vi "Read Write LS DAS App Config.vi"(7 "Write (F)":bool, 8 "Error IN":errorcluster, 10 "LS DAS Config":T1={"Location"="", "Profiles Path"=path "", "Current Profile"="", "CA Number"="", "Cycles Completed"=0, "Stagger Time (ms)"=0, "Pumps Present"={"Pump 1"=FALSE, "Pump 2"=FALSE, "Pump 3"=FALSE, "Pump 4"=FALSE, "Pump 5"=FALSE, "Pump 6"=FALSE}, "Data Log Init"={"Data Path"=path "", "Data Log Rate (S/s)"=0, "AKLH Rate (Hours/S)"=0.0, "Sync Time Offset (min)"=0, "IP Last 3"=0, "WebDAV IP"=""}, "Email Handler IP"="", "Cycle Threshold:"=3.0, "Cycle Pts to Avg:"=3, "Anomaly Threshold:"=3.0, "Normal Steps:"=3, "Step Threshold:"=3.0, "Bank 1 Offset"=0.0, "Bank 2 Offset"=0.0, "LS Power (Freq):"=0.0, "LS Power (Duty):"=0.0, "Bank 1 Present"={"1"=FALSE, "2"=FALSE, "3"=FALSE, "4"=FALSE, "5"=FALSE}, "Bank 2 Present"={"6"=FALSE, "7"=FALSE, "8"=FALSE, "9"=FALSE, "10"=FALSE}, "Data File Name"="", "Detection Mode"=0, "Serial Numbers"=[], "Profile Record"=FALSE, "Bank2 Record Rate"=0} {"Bank2 Record Rate" step=1; "Detection Mode" min=0 max=999999 step=1; "LS Power (Duty):" min=0.0 max=999999.0 step=1.0; "LS Power (Freq):" min=0.0 max=999999.0 step=1.0; "Bank 2 Offset" min=0.0 max=999999.0 step=1.0; "Bank 1 Offset" min=0.0 max=999999.0 step=1.0; "Step Threshold:" max=999999.0 step=1.0; "Normal Steps:" max=999999 step=1; "Anomaly Threshold:" max=999999.0 step=1.0; "Cycle Pts to Avg:" min=0 max=999999 step=1; "Cycle Threshold:" min=0.0 max=999999.0 step=1.0}, 11 "Refnum in":T3) -> (0 "Error OUT":errorcluster, 2 "LS DAS Config OUT":T1={"Location"="", "Profiles Path"=path "", "Current Profile"="", "CA Number"="", "Cycles Completed"=0, "Stagger Time (ms)"=0, "Pumps Present"={"Pump 1"=FALSE, "Pump 2"=FALSE, "Pump 3"=FALSE, "Pump 4"=FALSE, "Pump 5"=FALSE, "Pump 6"=FALSE}, "Data Log Init"={"Data Path"=path "", "Data Log Rate (S/s)"=0, "AKLH Rate (Hours/S)"=0.0, "Sync Time Offset (min)"=0, "IP Last 3"=0, "WebDAV IP"=""}, "Email Handler IP"="", "Cycle Threshold:"=3.0, "Cycle Pts to Avg:"=3, "Anomaly Threshold:"=3.0, "Normal Steps:"=3, "Step Threshold:"=3.0, "Bank 1 Offset"=0.0, "Bank 2 Offset"=0.0, "LS Power (Freq):"=0.0, "LS Power (Duty):"=0.0, "Bank 1 Present"={"1"=FALSE, "2"=FALSE, "3"=FALSE, "4"=FALSE, "5"=FALSE}, "Bank 2 Present"={"6"=FALSE, "7"=FALSE, "8"=FALSE, "9"=FALSE, "10"=FALSE}, "Data File Name"="", "Detection Mode"=0, "Serial Numbers"=[], "Profile Record"=FALSE, "Bank2 Record Rate"=0} {"Bank2 Record Rate" step=1; "Detection Mode" min=0 max=999999 step=1; "LS Power (Duty):" min=0.0 max=999999.0 step=1.0; "LS Power (Freq):" min=0.0 max=999999.0 step=1.0; "Bank 2 Offset" min=0.0 max=999999.0 step=1.0; "Bank 1 Offset" min=0.0 max=999999.0 step=1.0; "Step Threshold:" max=999999.0 step=1.0; "Normal Steps:" max=999999 step=1; "Anomaly Threshold:" max=999999.0 step=1.0; "Cycle Pts to Avg:" min=0 max=999999 step=1; "Cycle Threshold:" min=0.0 max=999999.0 step=1.0}, 3 "Refnum out":T3)   [LabVIEW 2018]
uses:
  <vilib>/Utility/config.llb/Config Data RefNum.ctl
  Type Defs/LS DAS App Config.ctl
  Data Logger/Data Log Init.ctl
  <vilib>/Utility/config.llb/NI_LVConfig.lvlib
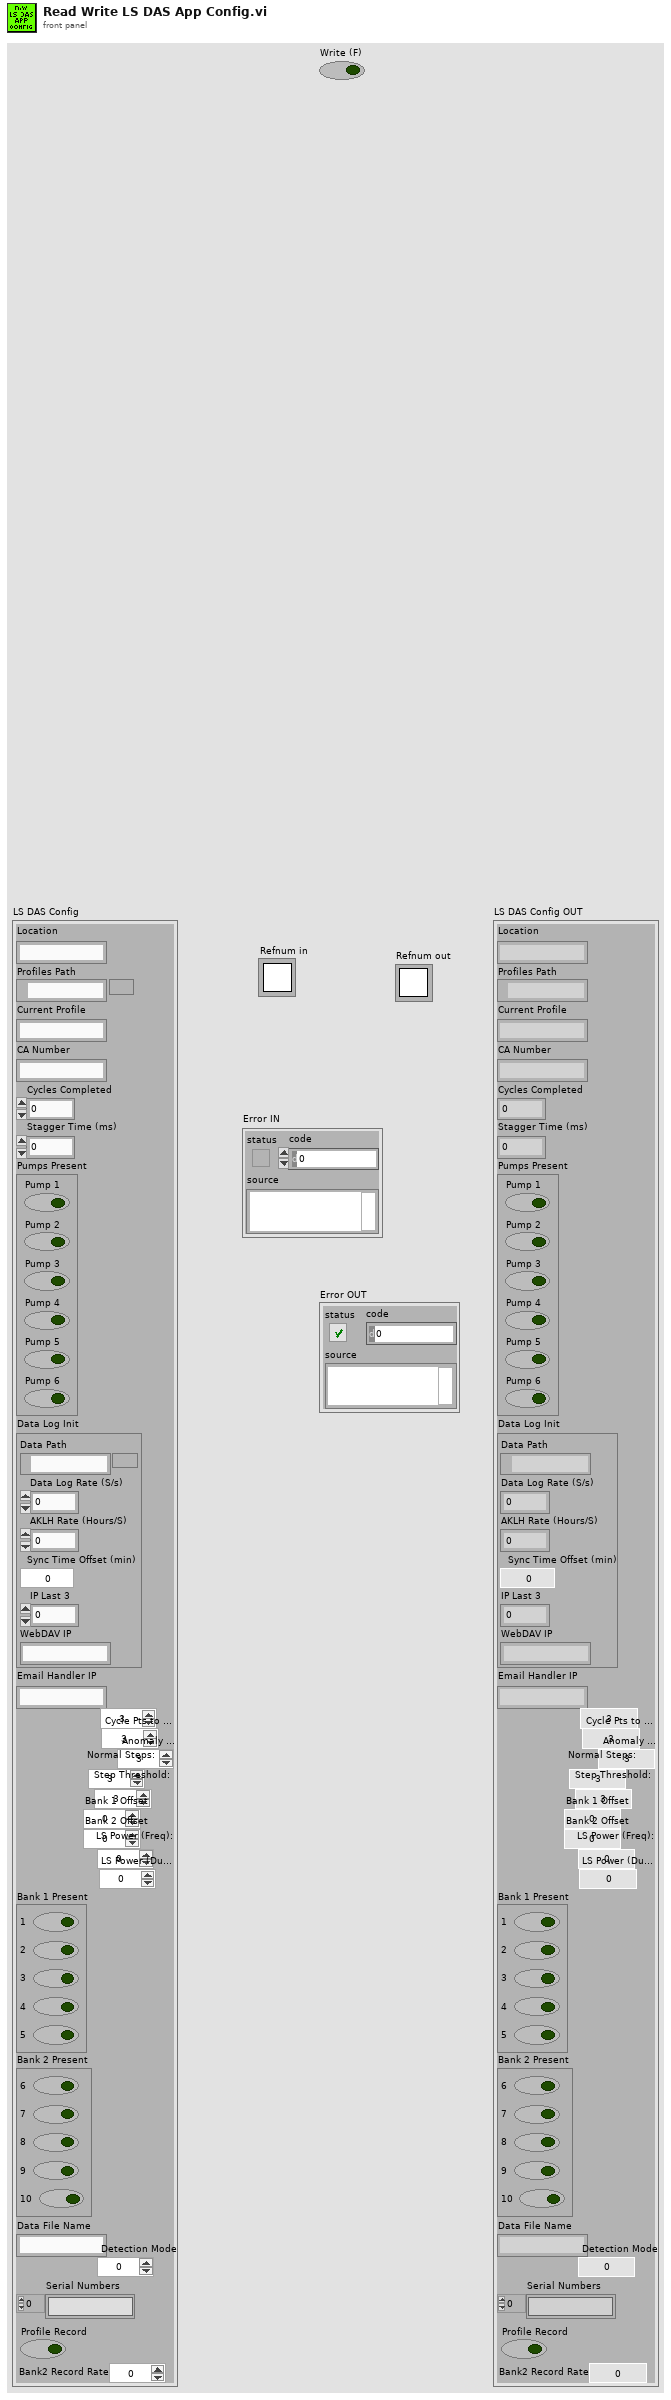
[diagram p1: front panel]
types:
  T1 = typedef "LS DAS App Config.ctl" = cluster{"Location":string, "Profiles Path":path, "Current Profile":string, "CA Number":string, "Cycles Completed":u32, "Stagger Time (ms)":i32, "Pumps Present":cluster{"Pump 1":bool, "Pump 2":bool, "Pump 3":bool, "Pump 4":bool, "Pump 5":bool, "Pump 6":bool}, "Data Log Init":T2, "Email Handler IP":string, "Cycle Threshold:":dbl, "Cycle Pts to Avg:":i32, "Anomaly Threshold:":dbl, "Normal Steps:":u32, "Step Threshold:":dbl, "Bank 1 Offset":dbl, "Bank 2 Offset":dbl, "LS Power (Freq):":dbl, "LS Power (Duty):":dbl, "Bank 1 Present":cluster{"1":bool, "2":bool, "3":bool, "4":bool, "5":bool}, "Bank 2 Present":cluster{"6":bool, "7":bool, "8":bool, "9":bool, "10":bool}, "Data File Name":string, "Detection Mode":i32, "Serial Numbers":string[], "Profile Record":bool, "Bank2 Record Rate":u16}
  T2 = typedef "Data Log Init.ctl" = cluster{"Data Path":path, "Data Log Rate (S/s)":u32, "AKLH Rate (Hours/S)":dbl, "Sync Time Offset (min)":i32, "IP Last 3":i32, "WebDAV IP":string}
  T3 = typedef "NI_LVConfig.lvlib/Config Data RefNum.ctl" = refnum<k1>
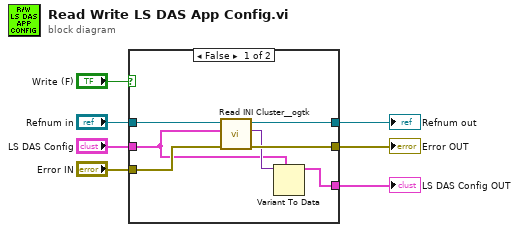
[diagram p0: block diagram]
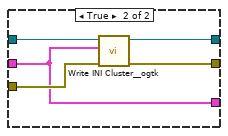
[diagram p2: hidden frame]
diagram:
  n1 = case shown="False" "Write (F)" {
    tunnel: "Refnum in" -> [w14 w19]
    tunnel: "LS DAS Config" -> [w10 w16]
    tunnel: "Error IN" -> [w13 w18]
    tunnel: [w8 w17] -> w4
    tunnel: [w9 w16] -> w1
    tunnel: [w12 w15] -> w5
    frame False {
      n2 = call <userlib>:"Read INI Cluster__ogtk.vi"("error in (no error)"=w13, "INI Fomatted Cluster Type"=w10, "refnum"=w14) -> ("error out"=w12:errorcluster, "INI Fomatted Cluster"=w11:variant, "dup refnum"=w8:T3)  [unwired: 4 in, 2 out]
      n3 = Variant To Data(type=w10, Variant=w11) -> (data=w9:T1)  [unwired: 1 in, 1 out]
    }
    frame True {
      n4 = call <userlib>:"Write INI Cluster__ogtk.vi"("error in (no error)"=w18, "INI Fomatted Cluster"=w16, "refnum"=w19) -> ("error out"=w15:errorcluster, "dup refnum"=w17:T3)  [unwired: 7 in]
    }
  }
  "Error OUT" <- w5
  "Refnum out" <- w4
  "LS DAS Config OUT" <- w1
